vi "FH_ErrorCase.vi"() -> ()   [LabVIEW 2016]
uses:
  <instrlib>/Zurich Instruments LabOne/Public/Configure/ziSetValueDouble.vi
  <instrlib>/Zurich Instruments LabOne/Zurich Instruments LabOne.lvlib
panel:
  out "error out 2":errorcluster
  in  "error out":errorcluster
  out "?":T1
  in  "freq":dbl=100.0
  in  "stop":bool
  out "freq":dbl
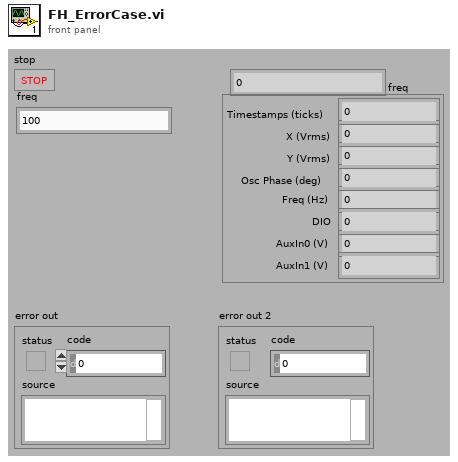
[diagram p1: front panel]
types:
  T1 = cluster{"Timestamps (ticks)":u64, "X (Vrms)":dbl, "Y (Vrms)":dbl, "Osc Phase (deg)":dbl, "Freq (Hz)":dbl, "DIO":u32, "AuxIn0 (V)":dbl, "AuxIn1 (V)":dbl}
  T2 = typedef "Zurich Instruments LabOne.lvlib/ziTypeHandle.ctl" = cluster{"handleValid":bool, "Conn":u64, "Path Prefix":string, "Handle":u64, "Connected":bool, "Clockbase(s)":dbl}
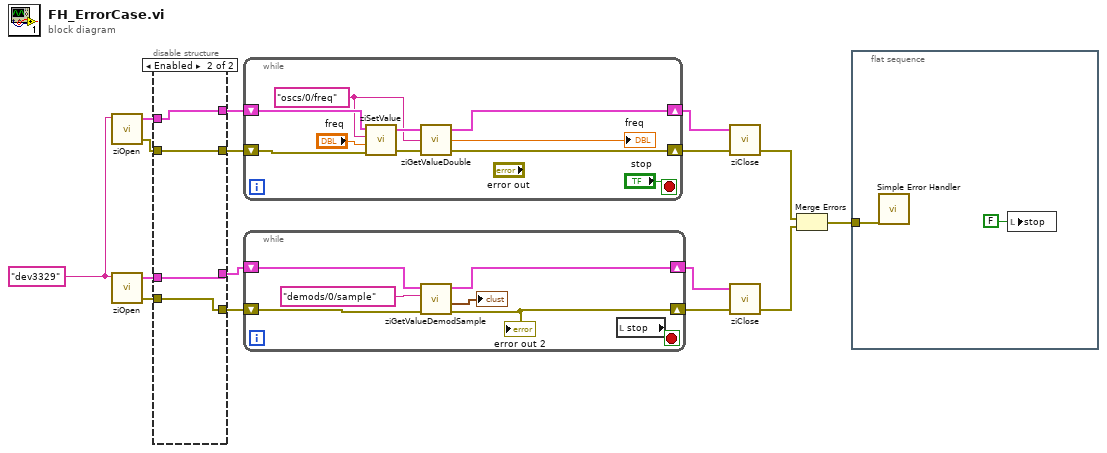
[diagram p0: block diagram]
diagram:
  w4 = "dev3329" ("Hostname obsolete (auto)")
  n1 = call <instrlib>:"ziOpen.vi"("Address"=w4) -> ("Error Out"=w9:errorcluster, "HandleOut"=w12:T2)  [unwired: 3 in, 1 out]
  n2 = call <instrlib>:"ziOpen.vi"("Address"=w4) -> ("Error Out"=w5:errorcluster, "HandleOut"=w7:T2)  [unwired: 3 in, 1 out]
  n3 = disable-structure shown="Enabled" {
    disable-tunnel: w12 -> [w19 w23]
    disable-tunnel: [w19 w23] -> w11
    disable-tunnel: [w18 w22] -> w10
    disable-tunnel: w9 -> [w18 w22]
    disable-tunnel: [w19 w21] -> w8
    disable-tunnel: w7 -> [_ w21]
    disable-tunnel: [w17 w20] -> w6
    disable-tunnel: w5 -> [w17 w20]
    frame Disabled {
    }
    frame Enabled {
    }
  }
  n4 = while {
    shift-right: [w26] -> w14
    shift-left: w10 -> [w28]
    shift-right: [w31] -> w16
    shift-left: w11 -> [w33]
    stop <- "stop" stop-if-true
    w30 = "oscs/0/freq" ("Path")
    n5 = call-poly <instrlib>:"ziSetValue.vi"("Error In"=w28, "Value"="freq", "Path"=w30, "Handle In"=w33) -> ("Error Out"=w27:errorcluster, "Handle Out"=w32:T2)  [unwired: 1 in]
    n6 = call <instrlib>:"ziGetValueDouble.vi"("error in"=w27, "Path"=w30, "Handle in"=w32) -> ("error out"=w26:errorcluster, "Value"=→"freq":dbl, "Handle out"=w31:T2)
  }
  n7 = while {
    shift-right: [w36] -> w13
    shift-left: w6 -> [w35]
    shift-right: [w38] -> w15
    shift-left: w8 -> [w39]
    stop <- w34 stop-if-true
    n8 = call <instrlib>:"ziGetValueDemodSample.vi"("error in"=w35, "Path"="demods/0/sample", "Handle In"=w39) -> ("error out"=w36:errorcluster, "Demod Sample Out"=→"?":T1, "Handle Out"=w38:T2)  [unwired: 2 in]
    "error out 2" <- w36
    n9 = local read "stop"() -> (w34:bool)
  }
  n10 = call <instrlib>:"ziClose.vi"("Error In"=w14, "Handle In"=w16) -> ("Error Out"=w3:errorcluster)  [unwired: 2 in, 1 out]
  n11 = call <instrlib>:"ziClose.vi"("Error In"=w13, "Handle In"=w15) -> ("Error Out"=w2:errorcluster)  [unwired: 2 in, 1 out]
  n12 = Merge Errors(w3, w2) -> (w1:errorcluster)
  n13 = flat-sequence {
    tunnel: w1 -> [w41]
    frame #0 {
      n14 = call <vilib>:"Simple Error Handler.vi"("error in (no error)"=w41) -> ()  [unwired: 4 in, 5 out]
      n15 = local write "stop"(FALSE ("stop")) -> ()
    }
  }
